vi "Get Array Type Descriptor.vi"(9 "error in (no error)":errorcluster, 10 ".NET AdsDataType":refnum<k24>) -> (1 "error out":errorcluster, 2 ".NET AdsDataType":refnum<k24>, 3 "Array Type Descriptor":T1={"Fundamental PLC Type"=enum."UNDEFINED", "Fundamental Type Byte Size"=0, "Item Count"=0, "Dimension Lengths"=[], "Sub-Item Type Descriptor"=variant(variant[] [])})   [LabVIEW 2018, in "TwinCAT ADS.lvclass"]
uses:
  TwinCAT ADS.lvclass
  TwinCAT.Ads
  Controls/PLC Array Type Descriptor.ctl
  Controls/PLC Type.ctl
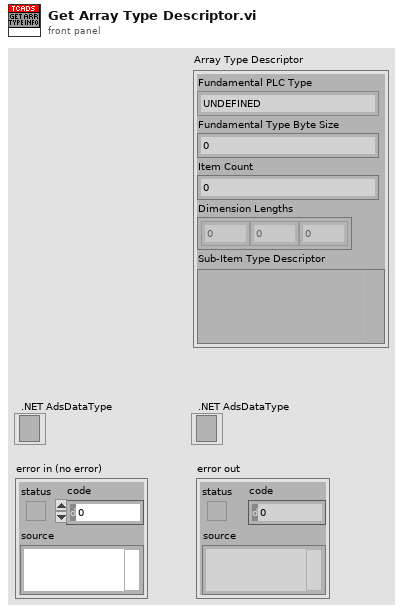
[diagram p1: front panel]
types:
  T1 = typedef "TwinCAT ADS.lvclass/PLC Array Type Descriptor.ctl" = cluster{"Fundamental PLC Type":T2, "Fundamental Type Byte Size":i32, "Item Count":i32, "Dimension Lengths":i32[], "Sub-Item Type Descriptor":variant}
  T2 = typedef "TwinCAT ADS.lvclass/PLC Type.ctl" = enum16{"UNDEFINED", "INT", "DINT", "REAL", "LREAL", "SINT", "BYTE", "UINT", "UDINT", "LINT", "ULINT", "STRING", "WSTRING", "BOOL", "TIME", "LTIME", "DATE", "DT", "TOD", "ARRAY", "JAGGED ARRAY", "STRUCT", "FUNCTION BLOCK", "POINTER", "USER DEFINED"}
  T3 = typedef "TwinCAT ADS.lvclass/PLC Sub-Item Type Descriptor.ctl" = cluster{"PLC Type":T2, "Offset":i32, "Byte Size":i32, "[Sub-Item/Array Type Descriptor]":variant[]}
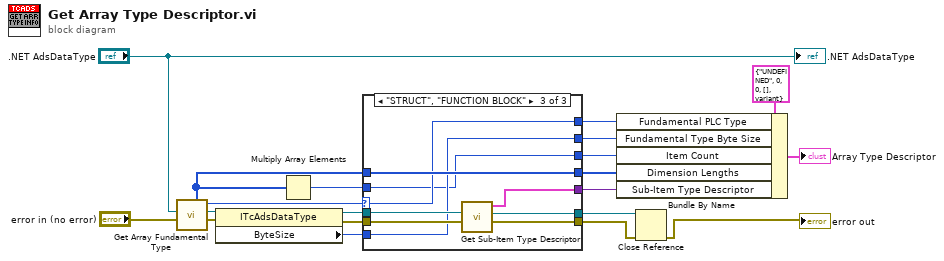
[diagram p0: block diagram]
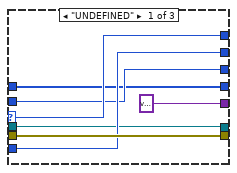
[diagram p2: hidden frame]
diagram:
  n1 = call "Get Array Fundamental Type.vi"("error in (no error)"="error in (no error)", ".NET AdsDataType"=".NET AdsDataType") -> ("error out"=w15:errorcluster, "Fundametal .NET AdsDataType"=w14:refnum<k24>, "Fundamental PLC Type"=w16:T2, "Dimension Lengths"=w12:i32[])  [unwired: 6 in]
  n2 = property class="ITcAdsDataType"(reference=w14, error in=w15) -> (reference out=w9:refnum<k24>, error out=w13:errorcluster, "ByteSize"=w10:i32)
  n3 = Multiply Array Elements(1:w12) -> (0:w11:i32)
  n4 = case shown="\"STRUCT\", \"FUNCTION BLOCK\"" w16 {
    selector: w16 -> [w26 w31 w37]
    tunnel: w13 -> [w27 w33 w41]
    tunnel: w12 -> [w23 w32 w42]
    tunnel: [w27 w33 w40] -> w2
    tunnel: w11 -> [w24 w29 w35]
    tunnel: w10 -> [w25 w30 w36]
    tunnel: w9 -> [w21 w28 w38]
    tunnel: [w26 w31 w37] -> w8
    tunnel: [w25 w30 w36] -> w7
    tunnel: [w24 w29 w35] -> w6
    tunnel: [w23 w32 w42] -> w5
    tunnel: [variant ("Variant") _ w39] -> w3
    tunnel: [w21 w28 w34] -> w1
    frame "UNDEFINED" {
    }
    frame Default {
    }
    frame "STRUCT", "FUNCTION BLOCK" {
      n5 = call "Get Sub-Item Type Descriptor.vi"("error in (no error)"=w41, ".NET AdsDataType"=w38) -> ("error out"=w40:errorcluster, ".NET AdsDataType"=w34:refnum<k24>, "[Sub-Item Type Descriptor]"=w39:T3[])  [unwired: 7 in]
    }
  }
  n6 = Bundle By Name(cluster=T1 {"Fundamental PLC Type"=enum."UNDEFINED", "Fundamental Type Byte Size"=0, "Item Count"=0, "Dimension Lengths"=[], "Sub-Item Type Descriptor"=variant(variant[] [])} ("Array Information"), "Fundamental PLC Type"=w8, "Fundamental Type Byte Size"=w7, "Item Count"=w6, "Dimension Lengths"=w5, "Sub-Item Type Descriptor"=w3) -> (→"Array Type Descriptor":T1)
  n7 = Close Reference(reference=w1, error in (no error)=w2) -> (error out=→"error out":errorcluster)
  ".NET AdsDataType" <- ".NET AdsDataType"
